vi "DummyDataSimulation.vi"() -> ()   [LabVIEW 2020]
uses:
  StateGPSUpdate.ctl
  <vilib>/Skyline/Message/NI Skyline Message.lvclass
  <vilib>/Skyline/Configuration/Configuration HTTP_class/NI Skyline Configuration HTTP.lvclass/NI Skyline Configuration HTTP.ctl
  TestData.ctl
  <vilib>/Skyline/Configuration/Configuration HTTP_class/Open Configuration HTTP.vi
  <vilib>/Skyline/Message/HTTP Wrapper/NI Skyline Message HTTP.lvclass
  C:/Program Files (x86)/National Instruments/LabVIEW 2020/vi.lib/Skyline/Message/NI Skyline Message.lvclass
  <vilib>/Skyline/Configuration/HTTP/Open Configuration (Desktop).vi
  <vilib>/Skyline/Message/HTTP Wrapper/Open (HTTP).vi
  <instrlib>/niSync/niSync.llb/niSync Read Last GPS or IRIG Timestamp (GPS).vi
  <vilib>/Skyline/Configuration/Configuration HTTP_class/NI Skyline Configuration HTTP.lvclass
  <vilib>/Skyline/Configuration/Configuration_class/NI Skyline Configuration.lvclass
  <vilib>/Skyline/Utilities/NI Skyline Utilities.lvlib
panel:
  in  "Test Drive Distance":dbl=1000.0
  out "Antenna Connected":bool
  out "Speed":dbl
  in  "SimulateOrHardware":bool
  in  "Resource Name":tag
  out "Percent Complete of Self Survey":i32
  out "Satellites Available":i32
  out "Mobile Mode":bool
  out "Latitude":dbl caption="latitude"
  out "Longitude":dbl caption="longitude"
  out "Altitude":dbl caption="altitude"
  in  "Stop":bool
  out "Current GPS Time":timestamp caption="time" format="%<%.9X\n%x>T"
  out "GPS time":timestamp
  out "timestamp":timestamp
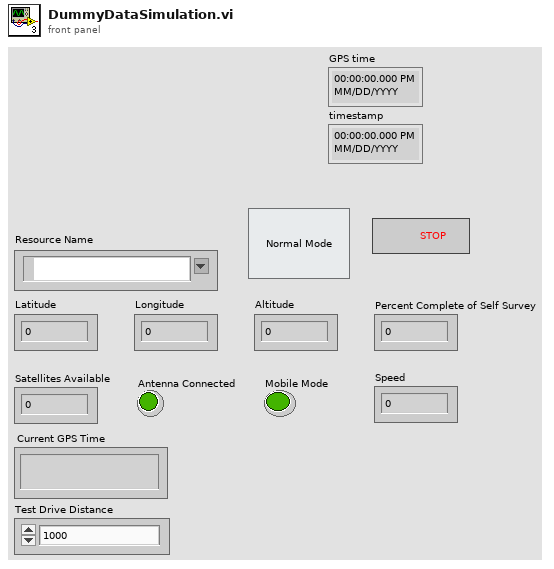
[diagram p1: front panel]
types:
  T1 = typedef "StateGPSUpdate.ctl" = enum16{"Init", "UpdateGPS", "Shutdown"}
  T2 = typedef "TestData.ctl" = cluster{"GPS":cluster{"Latitude":dbl, "Longitude":dbl, "Timestamp":string}, "SystemLinkClientInfo":cluster{"TargetName":string, "MinionID":string}, "CampaignData":cluster{"DistanceTraveled":dbl, "CampaignProgress":dbl, "Speed":dbl, "Moving":bool}}
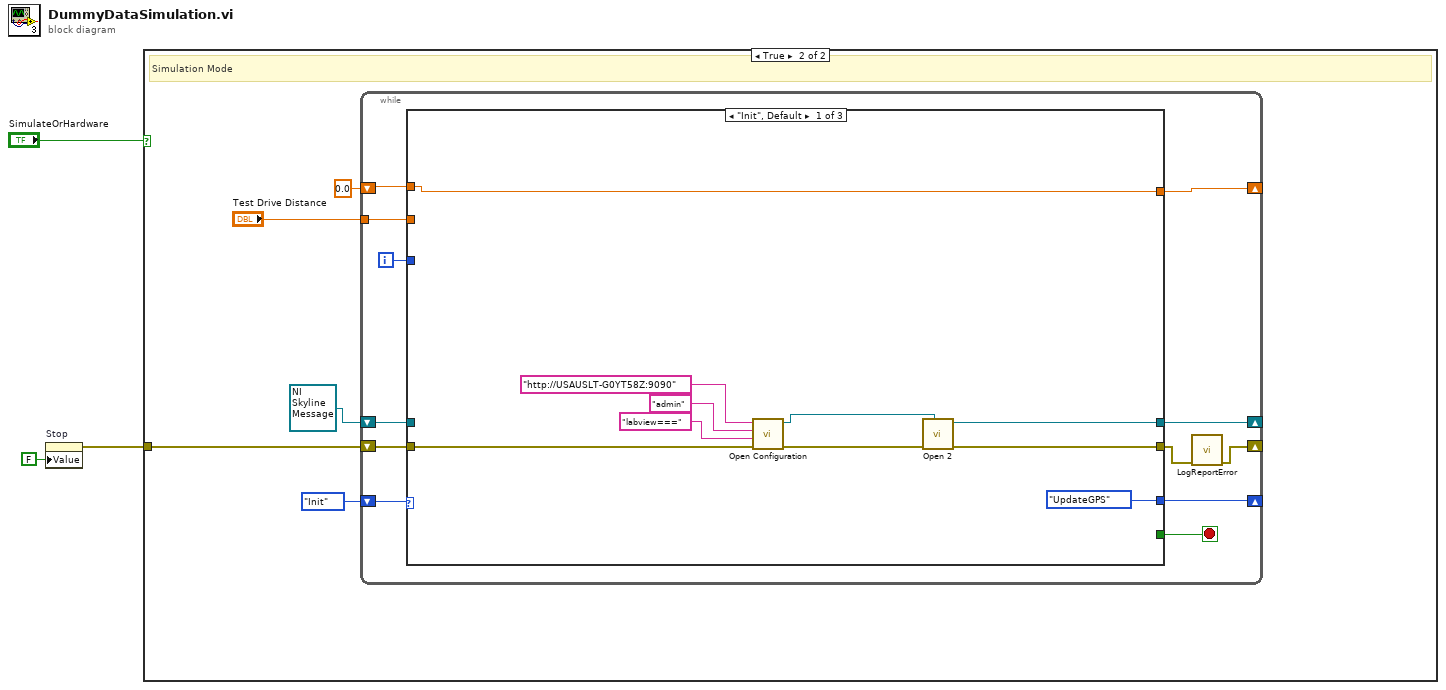
[diagram p0: block diagram]
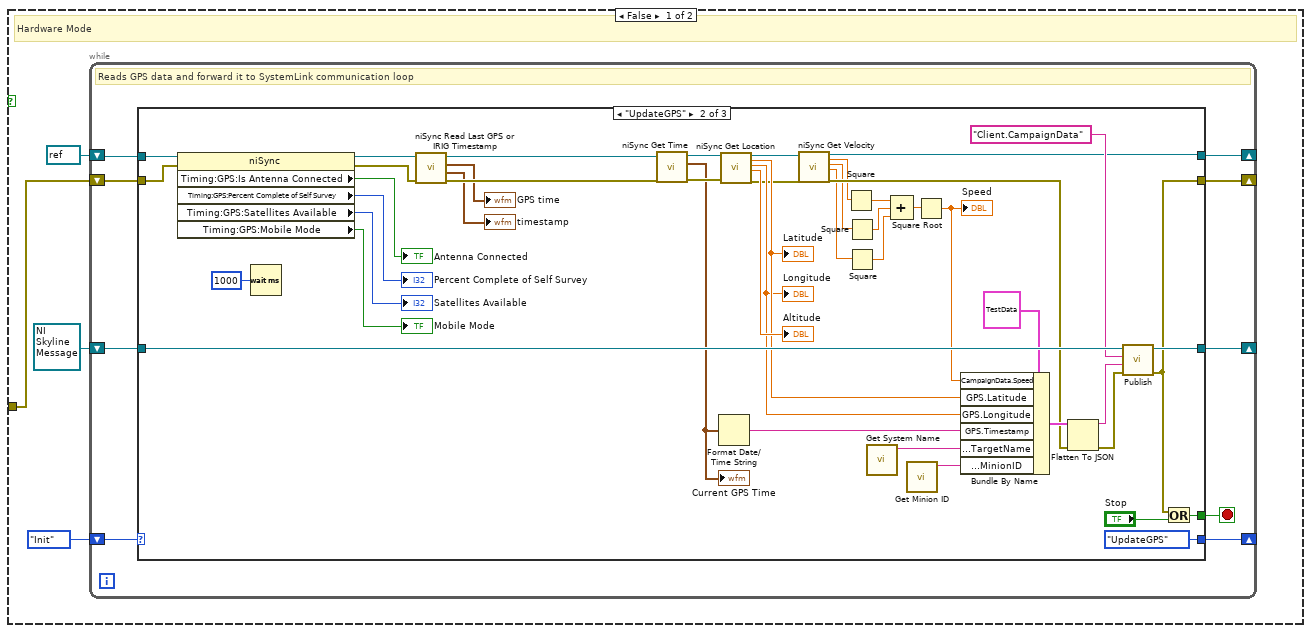
[diagram p2: hidden frame]
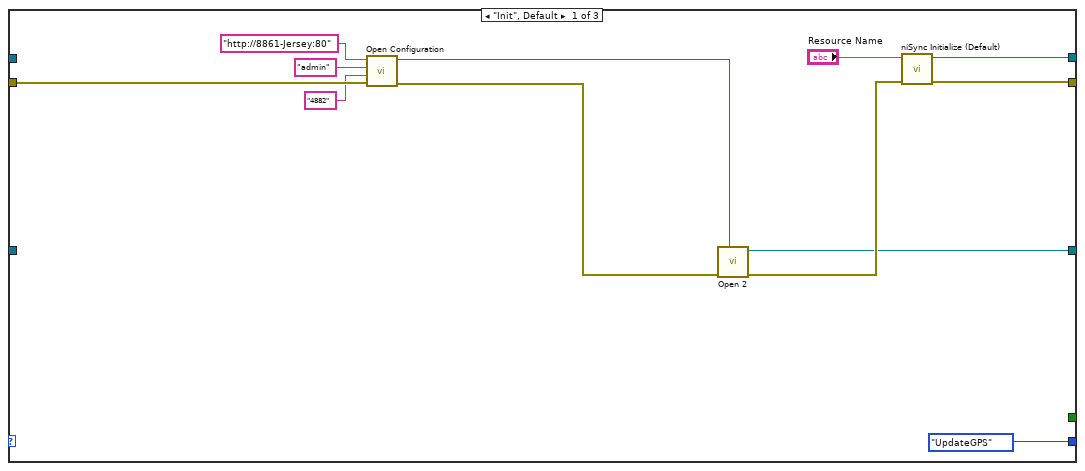
[diagram p3: hidden frame]
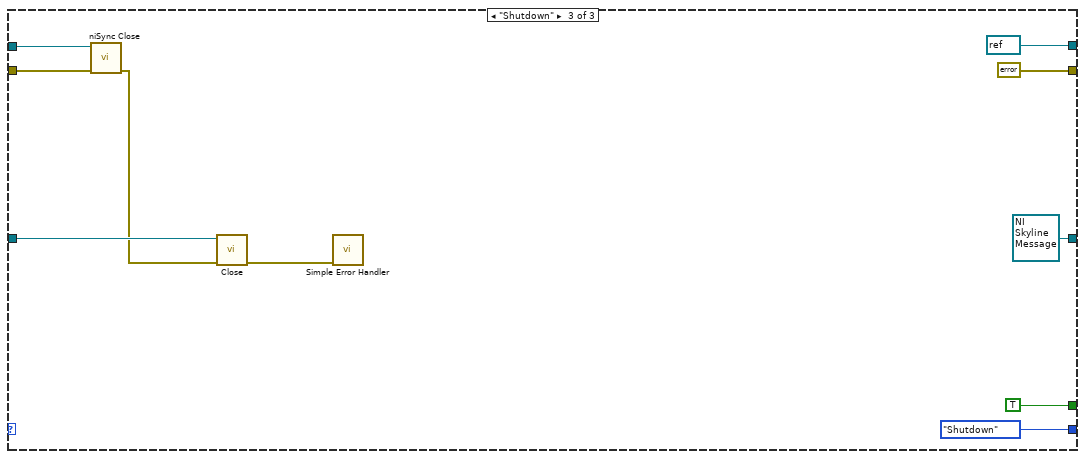
[diagram p4: hidden frame]
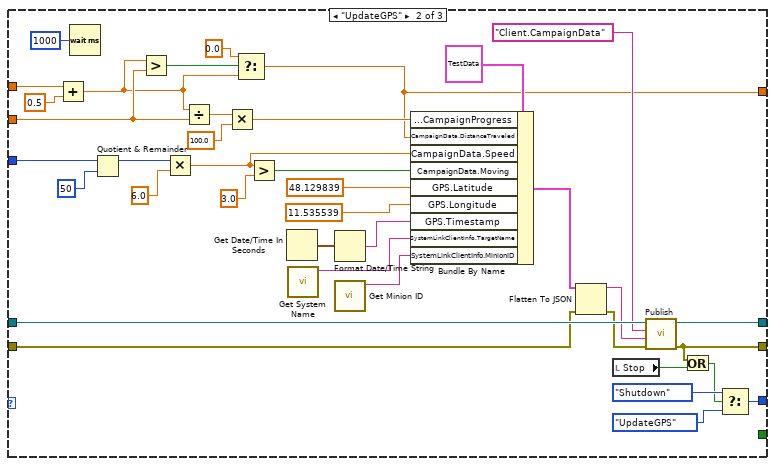
[diagram p5: hidden frame]
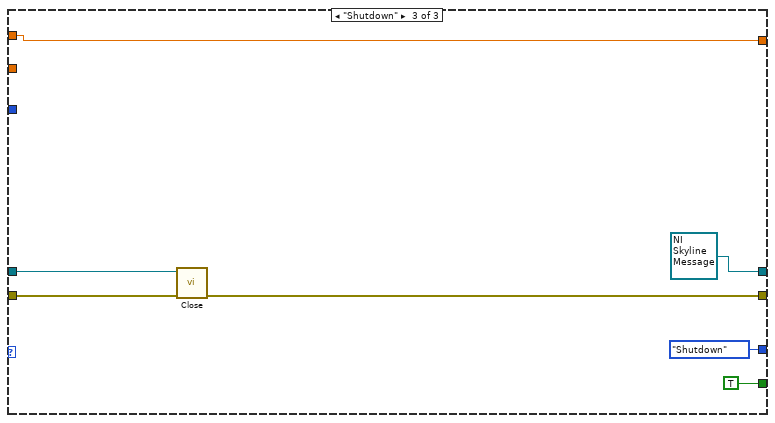
[diagram p6: hidden frame]
diagram:
  n1 = property on="Stop" class="Bool (strict)"("Value"=FALSE ("Stop")) -> (error out=w1:errorcluster)  [unwired: 2 in, 1 out]
  n2 = case shown="True" "SimulateOrHardware" {
    tunnel: w1 -> [w7 w87]
    frame False {
      # "Hardware Mode"
      n3 = while {
        shift-right: [w10] -> _
        shift-left: StateGPSUpdate."Init" -> [w11]
        shift-right: [w14] -> _
        shift-left: refnum<k15> refnum ("instrument handle out") -> [w16]
        shift-right: [w12] -> _
        shift-left: w7 -> [w15]
        shift-right: [w9] -> _
        shift-left: refnum<class "NI Skyline Message.lvclass"> refnum ("message session out") -> [w8]
        stop <- w13 stop-if-true
        # "Reads GPS data and forward it to SystemLink communication loop"
        n4 = case shown="\"UpdateGPS\"" w11 {
          tunnel: w16 -> [_ w73 w83]
          tunnel: w15 -> [w23 w58 w82]
          tunnel: [w27 w38 refnum<k15> refnum ("instrument handle out")] -> w14
          tunnel: [_ w69 TRUE] -> w13
          tunnel: [w26 w54 errorcluster {"status"=FALSE, "code"=0, "source"=""} ("error out")] -> w12
          tunnel: [StateGPSUpdate."UpdateGPS" StateGPSUpdate."UpdateGPS" StateGPSUpdate."Shutdown"] -> w10
          tunnel: [w17 w55 refnum<class "NI Skyline Message.lvclass"> refnum ("message session out")] -> w9
          tunnel: w8 -> [_ w56 w77]
          frame "Init", Default {
            n5 = call-poly <vilib>:"Open Configuration.vi"("error in (no error)"=w23, "password"="4882", "username"="admin", "server url"="http://8861-Jersey:80") -> ("error out"=w22:errorcluster, "configuration"=w18:refnum<class "NI Skyline Configuration HTTP.lvclass">)  [unwired: 6 in]
            n6 = call-poly <vilib>:"Open 2.vi"("configuration"=w18, "error in (no error)"=w22) -> ("error out"=w24:errorcluster, "message session"=w17:refnum<class "NI Skyline Message HTTP.lvclass">)  [unwired: 8 in]
            n7 = call <instrlib>:"niSync Initialize (Default).vi"("error in (no error)"=w24, "resource name"="Resource Name") -> ("error out"=w26:errorcluster, "instrument handle out"=w27:refnum<k15>)  [unwired: 8 in]
          }
          frame "UpdateGPS" {
            n8 = property class="niSync"(reference=w73, error in=w58) -> (reference out=w66:refnum<k15>, error out=w65:errorcluster, "Timing:GPS:Is Antenna Connected"=→"Antenna Connected":bool, "Timing:GPS:Percent Complete of Self Survey"=→"Percent Complete of Self Survey":i32, "Timing:GPS:Satellites Available"=→"Satellites Available":i32, "Timing:GPS:Mobile Mode"=→"Mobile Mode":bool)
            n9 = Wait (ms)(milliseconds to wait=u32 1000 ("millisecond multiple")) -> ()  [unwired: 1 out]
            n10 = call-poly <instrlib>:"niSync Read Last GPS or IRIG Timestamp.vi"("error in (no error)"=w65, "instrument handle"=w66) -> ("error out"=w63:errorcluster, "timestamp"=→"timestamp":timestamp, "GPS time"=→"GPS time":timestamp, "instrument handle out"=w64:refnum<k15>)  [unwired: 6 in]
            n11 = call <instrlib>:"niSync Get Time.vi"("error in (no error)"=w63, "instrument handle"=w64) -> ("error out"=w67:errorcluster, "time"=w42:timestamp, "instrument handle out"=w68:refnum<k15>)  [unwired: 5 in]
            "Current GPS Time" <- w42
            n12 = Format Date/Time String(seconds (now)=w42) -> (date/time string=w48:string)  [unwired: 2 in]
            n13 = call <instrlib>:"niSync Get Location.vi"("instrument handle"=w68, "error in (no error)"=w67) -> ("instrument handle out"=w40:refnum<k15>, "latitude"=w51:dbl, "longitude"=w50:dbl, "altitude"=→"Altitude":dbl, "error out"=w41:errorcluster)  [unwired: 13 in]
            "Latitude" <- w51
            "Longitude" <- w50
            n14 = call <instrlib>:"niSync Get Velocity.vi"("instrument handle"=w40, "error in (no error)"=w41) -> ("instrument handle out"=w38:refnum<k15>, "east velocity"=w36:dbl, "north velocity"=w35:dbl, "up velocity"=w37:dbl, "error out"=w39:errorcluster)  [unwired: 13 in]
            n15 = Square(x=w36) -> (x^2=w34:dbl)
            n16 = Square(x=w35) -> (x^2=w33:dbl)
            n17 = Square(x=w37) -> (x^2=w32:dbl)
            n18 = call <vilib>:"Get System Name.vi"() -> ("system name"=w47:string)  [unwired: 11 in]
            n19 = Compound Arithmetic op=ADD(w34, w33, w32) -> (w31:dbl)
            n20 = call <vilib>:"Get Minion ID.vi"() -> ("minion id"=w46:string)  [unwired: 11 in]
            n21 = Square Root(x=w31) -> (sqrt(x)=w30:dbl)
            "Speed" <- w30
            n22 = Bundle By Name(cluster=T2 {"GPS"={"Latitude"=0.0, "Longitude"=0.0, "Timestamp"=""}, "SystemLinkClientInfo"={"TargetName"="", "MinionID"=""}, "CampaignData"={"DistanceTraveled"=0.0, "CampaignProgress"=0.0, "Speed"=0.0, "Moving"=FALSE}}, "CampaignData.Speed"=w30, "GPS.Latitude"=w51, "GPS.Longitude"=w50, "GPS.Timestamp"=w48, "SystemLinkClientInfo.TargetName"=w47, "SystemLinkClientInfo.MinionID"=w46) -> (w45:T2)
            n23 = Flatten To JSON(anything=w45, error in (no error)=w39) -> (JSON string=w44:string, 11:w43:errorcluster)  [unwired: 1 in]
            n24 = call-dynamic "Publish.vi"("error in (no error)"=w43, "message"=w44, "topic"="Client.CampaignData", "message session in"=w56) -> ("error out"=w54:errorcluster, "message session out"=w55:refnum<class "NI Skyline Message.lvclass">)  [unwired: 6 in]
            n25 = Or(x=w54, y="Stop") -> (x .or. y?=w69:bool)
          }
          frame "Shutdown" {
            n26 = call <instrlib>:"niSync Close.vi"("error in (no error)"=w82, "instrument handle"=w83) -> ("error out"=w75:errorcluster)  [unwired: 9 in]
            n27 = call-dynamic "Close.vi"("error in (no error)"=w75, "message session"=w77) -> ("error out"=w74:errorcluster)  [unwired: 9 in]
            n28 = call <vilib>:"Simple Error Handler.vi"("error in (no error)"=w74) -> ()  [unwired: 4 in, 5 out]
          }
        }
      }
    }
    frame True {
      # "Simulation Mode"
      n29 = while {
        shift-right: [w89] -> _
        shift-left: w87 -> [w97]
        shift-right: [w98] -> _
        shift-left: StateGPSUpdate."Init" -> [w100]
        shift-right: [w99] -> _
        shift-left: refnum<class "NI Skyline Message.lvclass"> refnum ("message session out") -> [w95]
        tunnel: "Test Drive Distance" -> [w93]
        shift-right: [w92] -> _
        shift-left: 0.0 -> [w91]
        i -> [w94]
        stop <- w96 stop-if-true
        n30 = case shown="\"Init\", Default" w100 {
          tunnel: [w105 w148 w151] -> w90
          tunnel: [w104 w141 refnum<class "NI Skyline Message.lvclass"> refnum ("message session out")] -> w99
          tunnel: [StateGPSUpdate."UpdateGPS" w146 StateGPSUpdate."Shutdown"] -> w98
          tunnel: w97 -> [w102 w133 w152]
          tunnel: [_ _ TRUE] -> w96
          tunnel: w95 -> [_ w140 w153]
          tunnel: w94 -> [_ w120 _]
          tunnel: w93 -> [_ w115 _]
          tunnel: [w101 w111 w149] -> w92
          tunnel: w91 -> [w101 w124 w149]
          frame "Init", Default {
            n31 = call-poly <vilib>:"Open Configuration.vi"("error in (no error)"=w102, "password"="labview===", "username"="admin", "server url"="http://USAUSLT-G0YT58Z:9090") -> ("error out"=w106:errorcluster, "configuration"=w107:refnum<class "NI Skyline Configuration HTTP.lvclass">)  [unwired: 6 in]
            n32 = call-poly <vilib>:"Open 2.vi"("configuration"=w107, "error in (no error)"=w106) -> ("error out"=w105:errorcluster, "message session"=w104:refnum<class "NI Skyline Message HTTP.lvclass">)  [unwired: 8 in]
          }
          frame "UpdateGPS" {
            n33 = Add(x=w124, y=0.5) -> (x+y=w113:dbl)
            n34 = Wait (ms)(milliseconds to wait=u32 1000) -> ()  [unwired: 1 out]
            n35 = Quotient & Remainder(x=w120, y=50) -> (x-y*floor(x/y)=w117:i32)  [unwired: 1 out]
            n36 = Greater?(x=w113, y=w115) -> (0:w114:bool)
            n37 = Multiply(x=w117, y=6.0) -> (x*y=w116:dbl)
            n38 = Divide(x=w113, y=w115) -> (x/y=w127:dbl)
            n39 = Multiply(x=w127, y=100.0) -> (x*y=w125:dbl)
            n40 = Select(t=0.0, s=w114, f=w113) -> (s? t:f=w111:dbl)
            n41 = Greater?(x=w116, y=3.0) -> (0:w122:bool)
            n42 = Get Date/Time In Seconds() -> (seconds since 1Jan1904=w136:timestamp)
            n43 = call <vilib>:"Get System Name.vi"() -> ("system name"=w130:string)  [unwired: 11 in]
            n44 = Format Date/Time String(seconds (now)=w136) -> (date/time string=w135:string)  [unwired: 2 in]
            n45 = call <vilib>:"Get Minion ID.vi"() -> ("minion id"=w129:string)  [unwired: 11 in]
            n46 = Bundle By Name(cluster=T2 {"GPS"={"Latitude"=0.0, "Longitude"=0.0, "Timestamp"=""}, "SystemLinkClientInfo"={"TargetName"="", "MinionID"=""}, "CampaignData"={"DistanceTraveled"=0.0, "CampaignProgress"=0.0, "Speed"=0.0, "Moving"=FALSE}}, "CampaignData.CampaignProgress"=w125, "CampaignData.DistanceTraveled"=w111, "CampaignData.Speed"=w116, "CampaignData.Moving"=w122, "GPS.Latitude"=48.129839, "GPS.Longitude"=11.535539, "GPS.Timestamp"=w135, "SystemLinkClientInfo.TargetName"=w130, "SystemLinkClientInfo.MinionID"=w129) -> (w134:T2)
            n47 = Flatten To JSON(anything=w134, error in (no error)=w133) -> (JSON string=w137:string, 11:w132:errorcluster)  [unwired: 1 in]
            n48 = local read "Stop"() -> (w142:bool)
            n49 = call-dynamic "Publish.vi"("error in (no error)"=w132, "message"=w137, "topic"="Client.CampaignData", "message session in"=w140) -> ("error out"=w148:errorcluster, "message session out"=w141:refnum<class "NI Skyline Message.lvclass">)  [unwired: 6 in]
            n50 = Or(x=w148, y=w142) -> (x .or. y?=w143:bool)
            n51 = Select(t=StateGPSUpdate."Shutdown", s=w143, f=StateGPSUpdate."UpdateGPS") -> (s? t:f=w146:T1)
          }
          frame "Shutdown" {
            n52 = call-dynamic "Close.vi"("error in (no error)"=w152, "message session"=w153) -> ("error out"=w151:errorcluster)  [unwired: 9 in]
          }
        }
        n53 = call "LogReportError.vi"("error in (no error)"=w90) -> ("error out"=w89:errorcluster)  [unwired: 10 in]
      }
    }
  }
